vi "Control Arm Sholder with PID 2.vi"(3 "stop":bool) -> (0 "busy":bool, 1 "motorStop":bool)   [LabVIEW 2015]
uses:
  <vilib>/myRIO/Common/Instrument Driver Framework/myRIO v1.0/Encoder/typedefs/Encoder Signal Mode.ctl
  <vilib>/myRIO/Instrument Drivers/Onboard IO/Encoder/typedefs/Encoder Reference.ctl
  <vilib>/myRIO/Common/Instrument Driver Framework/Utilities/typedefs/myRIO Generic Hardware Reference.ctl
  <vilib>/myRIO/Common/Instrument Driver Framework/Utilities/typedefs/Hardware Version Enum.ctl
  <vilib>/myRIO/Common/Instrument Driver Framework/Utilities/typedefs/myRIO v1.0 Reference.ctl
  <vilib>/myRIO/Common/Instrument Driver Framework/Utilities/typedefs/Generic FPGA Reference.ctl
  <vilib>/myRIO/Common/Instrument Driver Framework/myRIO v1.0/Encoder/typedefs/Encoder Channels Enum.ctl
  <vilib>/myRIO/Common/Instrument Driver Framework/myRIO v1.0/Encoder/typedefs/Encoder Configuration v1.0.ctl
  <vilib>/userdefined/High Color/nirio_resource_hc.ctl
  <vilib>/myRIO/Common/Instrument Driver Framework/Utilities/vis/Is FPGA Ref Available.vi
  <vilib>/myRIO/Common/Instrument Driver Framework/myRIO v1.0/Encoder/vis/myRIO v1.1 Open Encoder.vi
  <vilib>/myRIO/Instrument Drivers/Onboard IO/Encoder/vis/Read.vi
  <vilib>/myRIO/Common/Instrument Driver Framework/Utilities/vis/Validate Channels.vi
  <vilib>/myRIO/Common/Instrument Driver Framework/myRIO v1.0/Encoder/vis/myRIO v1.0 Reserve Encoder.vi
  <vilib>/myRIO/Common/Instrument Driver Framework/myRIO v1.0/Encoder/vis/myRIO v1.0 Build MUX Configuration Encoder.vi
  <vilib>/myRIO/Common/Instrument Driver Framework/myRIO v1.0/Resource Manager/vis/myRIO v1.0 Reserve Channel List.vi
  <vilib>/myRIO/Common/Instrument Driver Framework/myRIO v1.0/Resource Manager/vis/myRIO v1.0 Create Configuration List.vi
  <vilib>/myRIO/Common/Instrument Driver Framework/myRIO v1.0/Resource Manager/vis/myRIO v1.0 Reserve Channel.vi
  <vilib>/myRIO/Common/Instrument Driver Framework/myRIO v1.0/Resource Manager/vis/myRIO v1.0 Unreserve Channel.vi
  <vilib>/myRIO/Common/Instrument Driver Framework/myRIO v1.0/Resource Manager/vis/myRIO v1.0 Build Mutex Name.vi
  Global Angle.vi
  <vilib>/Utility/VariantDataType/GetNumericInfo.vi
  <vilib>/Utility/error.llb/Error Cluster From Error Code.vi
  <vilib>/myRIO/Common/Instrument Driver Framework/myRIO v1.0/myRIO v1.1 Open.vi
  <vilib>/myRIO/Common/Instrument Driver Framework/Utilities/vis/IO Manager.vi
  <vilib>/myRIO/Common/Instrument Driver Framework/Utilities/vis/Configuration Manager.vi
  <vilib>/myRIO/Common/Instrument Driver Framework/myRIO v1.0/Resource Manager/vis/myRIO v1.0 Configure IO.vi
  <vilib>/myRIO/Common/Instrument Driver Framework/myRIO v1.0/myRIO v1.0 Close.vi
  <vilib>/myRIO/Common/Instrument Driver Framework/myRIO v1.0/Encoder/vis/myRIO v1.0 Configure Encoder.vi
  <vilib>/myRIO/Common/Instrument Driver Framework/myRIO v1.0/Encoder/vis/myRIO v1.0 Read Encoder.vi
  <vilib>/myRIO/Express VI/Onboard IO/Encoder/Encoder Express VI.xnode
  <vilib>/myRIO/Instrument Drivers/Onboard IO/Encoder/vis/myRIO Encoder Open.xnode
  <vilib>/myRIO/Common/Instrument Driver Framework/myRIO v1.0/Encoder/typedefs/Encoder Count Direction Enum.ctl
  <vilib>/myRIO/Instrument Drivers/Onboard IO/Encoder/Encoder.lvlib
panel:
  out "output variable":sgl
  out "x = y? 3":bool
  out "x = y? 2":bool
  out "x = y?":bool
  out "differential":i32
  out "error":i32
  out "Input Rotations":dbl
  out "lastError":dbl
  out "integral":dbl
  out "Counter Value":i32
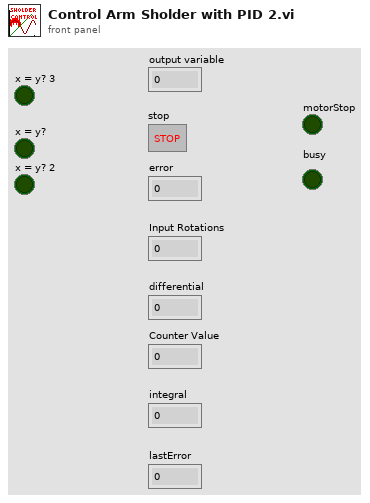
[diagram p1: front panel]
types:
  T1 = typedef "Encoder.lvlib/Encoder Reference.ctl" = cluster{"myRIO Reference":T2, "Encoder Channels Enum":T6}
  T2 = typedef "myRIO Generic Hardware Reference.ctl" = cluster{"myRIO Model":T3, "myRIO Hardware Reference":T4}
  T3 = typedef "Hardware Version Enum.ctl" = enum16{"Unknown", "myRIO-1900", "myRIO-1950", "roboRIO"}
  T4 = typedef "myRIO v1.0 Reference.ctl" = cluster{"Generic FPGA Reference":T5, "Allow multiple opens":bool}
  T5 = typedef "Generic FPGA Reference.ctl" = refnum<k20>
  T6 = typedef "Encoder Channels Enum.ctl" = enum16{"Not Connected", "C/ENC0", "C/ENC1", "A/ENC", "B/ENC", "DIO/ENC0", "DIO/ENC1", "DIO/ENC2", "DIO/ENC3", "DIO/ENC4"}
  T7 = typedef "Encoder Signal Mode.ctl" = enum16{"Quadrature phase signal", "Step and direction signal"}
  T8 = typedef "nirio_resource_hc.ctl" = tag
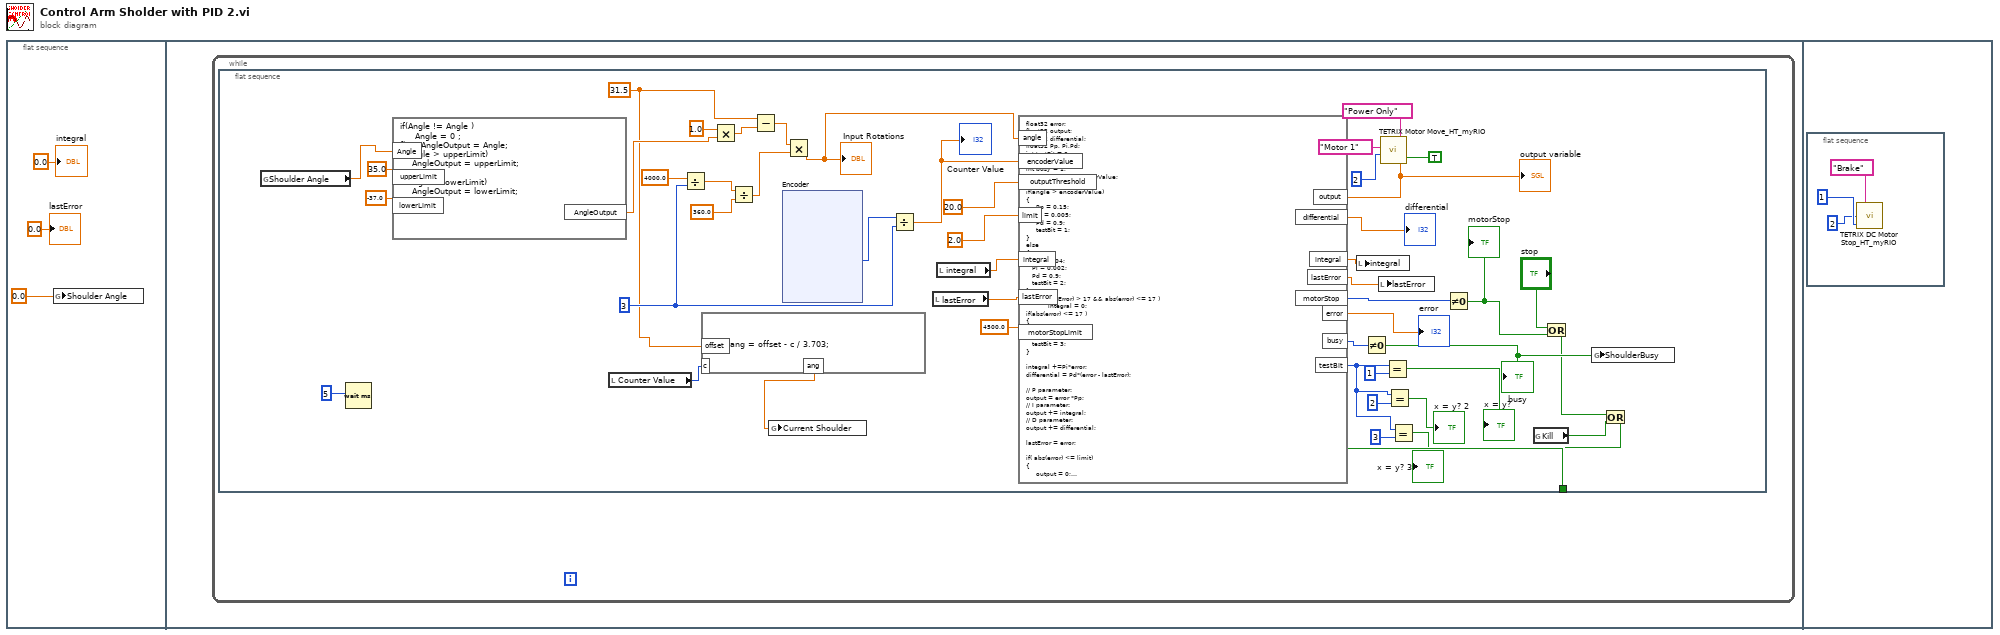
[diagram p0: block diagram]
diagram:
  n1 = flat-sequence {
    frame #0 {
      n2 = global write "Global Angle.vi" "Shoulder Angle"(0.0 ("angle")) -> ()
      "integral" <- 0.0 ("integral")
      "lastError" <- 0.0 ("lastError")
    }
    frame #1 {
      n3 = while {
        stop <- w4 stop-if-true
        n4 = flat-sequence {
          tunnel: [w6] -> w4
          frame #0 {
            w8 = 31.5 ("y")
            w17 = 3 ("y")
            n5 = global read "Global Angle.vi" "Shoulder Angle"() -> (w11:dbl)
            n6 = Wait (ms)(milliseconds to wait=u32 5 ("millisecond multiple")) -> ()  [unwired: 1 out]
            n7 = formula code="if(Angle != Angle )\n     Angle = 0 ;\nfloat AngleOutput = Angle;\nif(Angle > upperLimit)\n    AngleOutput = upperLimit;\n\nif(Angle < lowerLimit)\n    AngleOutput = lowerLimit;"("Angle"=w11, "upperLimit"=35.0 ("input variable"), "lowerLimit"=-37.0 ("input variable")) -> ("AngleOutput"=w29:dbl)
            n8 = local read "Counter Value"() -> (w10:i32)
            n9 = Divide(x=4000.0, y=w17) -> (x/y=w19:dbl)
            n10 = formula code="float ang = offset - c / 3.703;"("c"=w10, "offset"=w8) -> ("ang"=w9:dbl)
            n11 = Multiply(x=1.0, y=w29) -> (x*y=w34:dbl)
            n12 = Divide(x=w19, y=360.0) -> (x/y=w21:dbl)
            n13 = Subtract(x=w8, y=w34) -> (x-y=w35:dbl)
            n14 = global write "Global Angle.vi" "Current Shoulder"(w9) -> ()
            n15 = xnode "Encoder"() -> ("Counter Value"=w44:i32)  [unwired: 2 in, 3 out]
            n16 = Multiply(x=w35, y=w21) -> (x*y=w23:dbl)
            "Input Rotations" <- w23
            n17 = Divide(x=w44, y=w17) -> (x/y=w43:dbl)
            "Counter Value" <- w43
            n18 = local read "lastError"() -> (w46:dbl)
            n19 = local read "integral"() -> (w47:dbl)
            n20 = formula code="float32 error;\nfloat32 output;\nfloat32 differential;\nfloat32 Pp, Pi,Pd;\nint testBit = 0;\nint motorStop = 0;\nint busy = 1;\nerror = angle - encoderValue;\n\nif(angle > encoderValue)\n{\n     Pp = 0.15;\n     Pi = 0.005;\n     Pd = 0.9;\n     testBit = 1;\n}\nelse\n{\n   Pp = 0.04;\n   Pi = 0.002;\n   Pd = 0.9;\n   testBit = 2;\n}\nif( abs(lastError) > 17 && abs(error) <= 17 )\n           integral = 0;\nif(abs(error) <= 17 )\n{\n   Pi *= 30;\n   Pp *= 5;\n   testBit = 3;\n}\n        \nintegral +=Pi*error;\ndifferential = Pd*(error - lastError);\n\n// P parameter:\noutput = error *Pp;\n// I parameter:\noutput += integral;\n// D parameter:\noutput += differential;\n\nlastError = error;\n\nif( abs(error) <= limit)\n{\n     output = 0;\n      integral = 0;\n      busy = 0;\n}\n \n\nif( abs(output) >= outputThreshold)\n {\n      if(output > 0)\n                   output = outputThreshold;\n      else \n                  output = -1*outputThreshold;\n}\n\n\n\nif(abs(integral) >= motorStopLimit && abs(error) <= 17 )\n      motorStop = 1;"("angle"=w23, "encoderValue"=w43, "outputThreshold"=20.0 ("input variable"), "limit"=2.0 ("input variable"), "integral"=w47, "lastError"=w46, "motorStopLimit"=4500.0 ("input variable")) -> ("output"=w20:sgl, "integral"=w48:dbl, "lastError"=w45:dbl, "error"=→"error":sgl, "motorStop"=w41:i32, "differential"=→"differential":sgl, "busy"=w36:i32, "testBit"=w13:i32)
            "output variable" <- w20
            n21 = local write "integral"(w48) -> ()
            n22 = Not Equal To 0?(x=w36) -> (x != 0?=w15:bool)
            "busy" <- w15
            n23 = local write "lastError"(w45) -> ()
            n24 = call <vilib>:"TETRIX Motor Move_HT_myRIO.vi"("Power (-100 to 100)\n0 = Stop/Brake\n-128 = Stop/Coast"=w20, "Reverse? : T or F"=TRUE, "Control Mode"="Power Only", "Controller Daisy Chain Position: 1 - 4"=u8 2, "Select Channel"="Motor 1") -> ()  [unwired: 2 in, 1 out]
            n25 = Equal?(x=w13, y=1) -> (x = y?=→"x = y?":bool)
            n26 = Equal?(x=w13, y=2) -> (x = y?=→"x = y? 2":bool)
            n27 = Equal?(x=w13, y=3) -> (x = y?=→"x = y? 3":bool)
            n28 = Not Equal To 0?(x=w41) -> (x != 0?=w16:bool)
            "motorStop" <- w16
            n29 = global read "Global Angle.vi" "Kill"() -> (w5:bool)
            n30 = Or(x="stop", y=w16) -> (x .or. y?=w7:bool)
            n31 = global write "Global Angle.vi" "ShoulderBusy"(w15) -> ()
            n32 = Or(x=w7, y=w5) -> (x .or. y?=w6:bool)
          }
        }
      }
    }
    frame #2 {
      n33 = flat-sequence {
        frame #0 {
          n34 = call <vilib>:"TETRIX DC Motor Stop_HT_myRIO.vi"("Stop (Brake or Coast)"="Brake", "Motor Channel: (1 or 2)"=u8 1, "Controller Daisy Chain Position: 1 - 4"=u8 2) -> ()  [unwired: 1 in, 1 out]
        }
      }
    }
  }
